vi "trapezoidal.vi"() -> ()   [LabVIEW 2017]
uses:
  <vilib>/Analysis/1siggen.llb/Ramp Pattern by Samples.vi
  <vilib>/Analysis/NI_AALBase.lvlib
panel:
  in  "%Baixo":dbl
  out "Waveform Graph":dbl[](graph)
  in  "%Descida":dbl
  in  "%Alto":dbl
  in  "%Subida":dbl
  in  "Amplitude":dbl
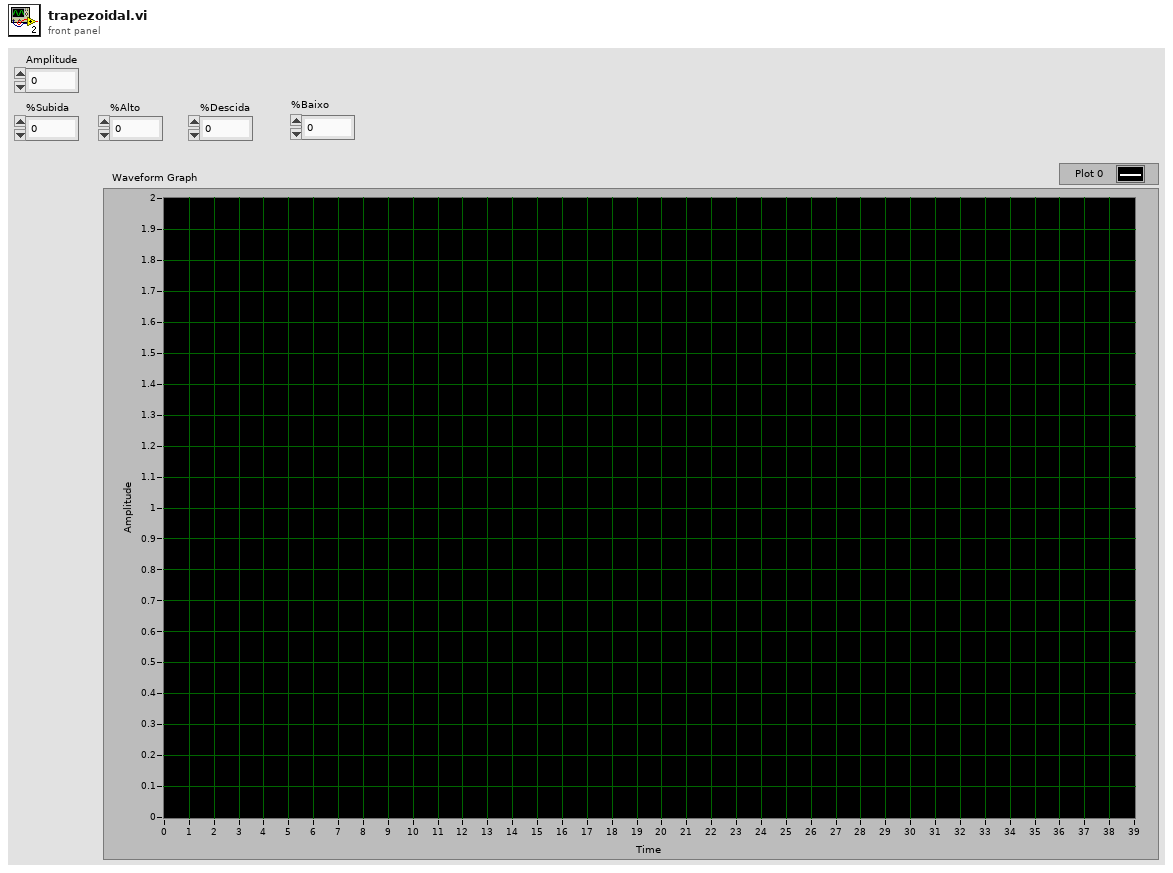
[diagram p1: front panel]
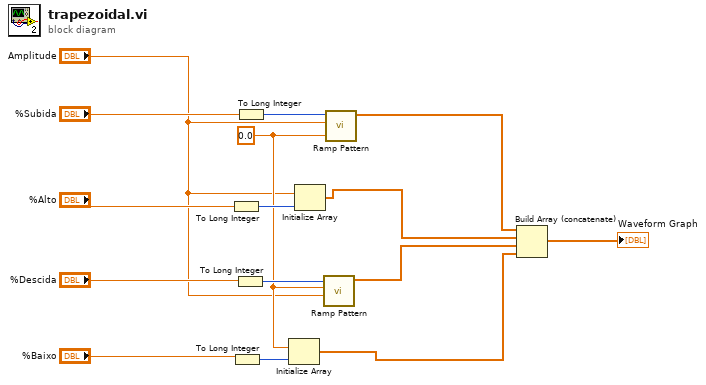
[diagram p0: block diagram]
diagram:
  w2 = 0.0 ("start")
  n1 = To Long Integer(number="%Alto") -> (32bit integer=w10:i32)
  n2 = To Long Integer(number="%Baixo") -> (32bit integer=w8:i32)
  n3 = To Long Integer(number="%Descida") -> (32bit integer=w14:i32)
  n4 = To Long Integer(number="%Subida") -> (32bit integer=w15:i32)
  n5 = Initialize Array(w2, w8) -> (w7:dbl[])
  n6 = Initialize Array("Amplitude", w10) -> (w9:dbl[])
  n7 = call-poly <vilib>:"Ramp Pattern.vi"("start"="Amplitude", "end"=w2, "samples"=w14) -> ("Ramp Pattern"=w11:dbl[])  [unwired: 7 in, 1 out]
  n8 = call-poly <vilib>:"Ramp Pattern.vi"("start"=w2, "end"="Amplitude", "samples"=w15) -> ("Ramp Pattern"=w12:dbl[])  [unwired: 7 in, 1 out]
  n9 = Build Array (concatenate)(w12, w9, w11, w7) -> (→"Waveform Graph":dbl[])
